vi "ble_cmd_gap_discover.vi"(8 "error in (no error)":errorcluster, 10 "GAP Discover Mode (Generic)":T1=1 items=["Discover Limited", "Discover Generic", "Discover Observation"], 11 "COM Bluegiga in":refnum<visa-resource-name>) -> (0 "error out":errorcluster, 3 "COM Bluegiga out":refnum<visa-resource-name>)   [LabVIEW 2017]
uses:
  type_def/gap_discover_mode.ctl
  type_def/message_class.ctl
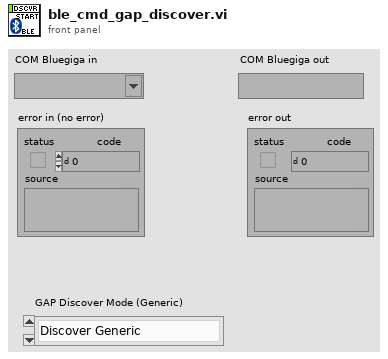
[diagram p1: front panel]
types:
  T1 = typedef "gap_discover_mode.ctl" = u8
  T2 = typedef "message_class.ctl" = u8
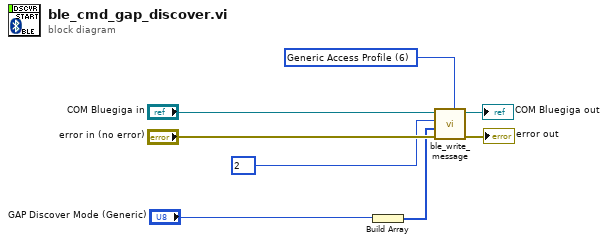
[diagram p0: block diagram]
diagram:
  w4 = T2 6 items=["System", "Persistent Store", "Attribute database", "Connection", "Attribute client", "Security Manager", "Generic Access Profile", "Hardware"] ("Command Class (System)")
  n1 = Build Array("GAP Discover Mode (Generic)") -> (w5:T1[])
  n2 = call "ble_write_message.vi"("Command Class (System)"=w4, "error in (no error)"="error in (no error)", "Payload(Empty)"=w5, "Message ID (0x00)"=u8 2, "COM Bluegiga in"="COM Bluegiga in") -> ("error out"=→"error out":errorcluster, "COM Bluegiga out"=→"COM Bluegiga out":refnum<visa-resource-name>)  [unwired: 4 in, 1 out]
